vi "Error_pop-up.vi"(1 "New msg":string, 2 "Mode":bool) -> ()   [LabVIEW 2011]
panel:
  out "Message":string
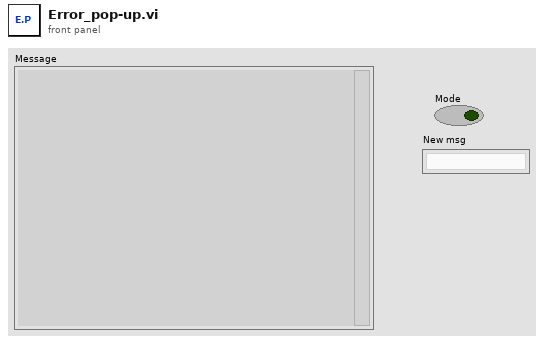
[diagram p1: front panel]
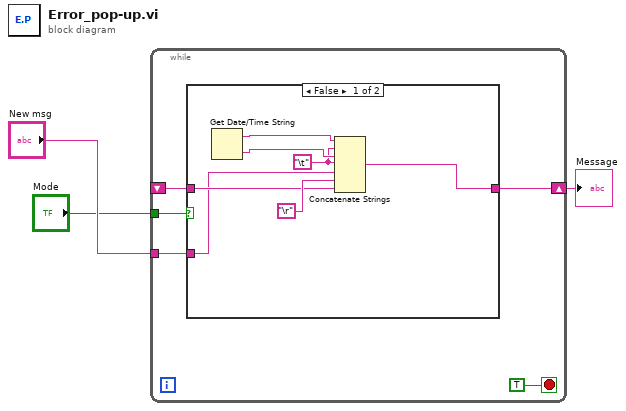
[diagram p0: block diagram]
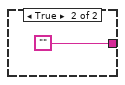
[diagram p2: hidden frame]
diagram:
  n1 = while {
    shift-right: [w8] -> w2
    shift-left: _ -> [w6]
    tunnel: "New msg" -> [w5]
    tunnel: "Mode" -> [w4]
    stop <- TRUE stop-if-true
    n2 = case shown="False" w4 {
      tunnel: [w14 ""] -> w8
      tunnel: w6 -> [w13 _]
      tunnel: w5 -> [w12 _]
      frame False {
        w9 = "\t"
        n3 = Get Date/Time String() -> (date string=w11:string, time string=w10:string)  [unwired: 3 in]
        n4 = Concatenate Strings(w11, w9, w10, w9, w12, "\r", w13) -> (w14:string)
      }
      frame True {
      }
    }
  }
  "Message" <- w2
